vi "Error Create Queue.vi"(8 "error in (no error)":errorcluster) -> (0 "error out":errorcluster, 2 "Error Queue out":refnum<queue>, 3 "Error out":refnum<class "Error.lvclass">)   [LabVIEW 2019, in "TSC Error.lvlib"]
doc: "This VI will obtain a reference to the TSC Error Queue. If has not already been created, it will create the Queue.\n\nInputs:\n-error in\n\nOutputs:\n-Error out [obj] - the error class output\n-Error Queue out [Queue Ref] - a reference to the Error queue\n-error out\n________________________________________________________________________________\n<b>Code Developed By:</b>\nDaniel Coons\nTechnology Service Corporation\n1983 S Liberty Drive\nBloomington, IN 47403\nPhone: 812 558-7100\ndaniel.coons@tsc.com\nwww.tsc.com\n\n<b>Date Created:</b> 11 AUG 2014\n<b>Date Updated:</b>"
uses:
  TSC Error.lvlib
  _Messages/Error/Error.lvclass
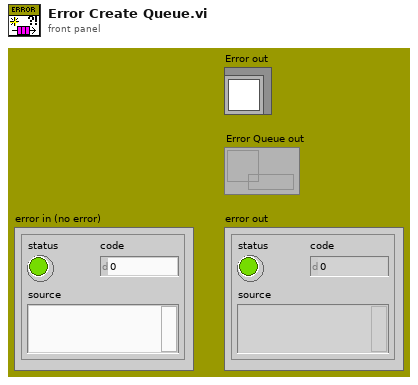
[diagram p1: front panel]
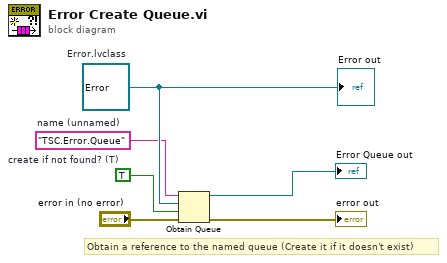
[diagram p0: block diagram]
diagram:
  w6 = refnum<class "Error.lvclass"> refnum  # Error.lvclass
  w5 = TRUE  # create if not found? (T)
  w3 = "TSC.Error.Queue"  # name (unnamed)
  # "Obtain a reference to the named queue (Create it if it doesn't exist)"
  n1 = Obtain Queue(name (unnamed)=w3, element data type=w6, create if not found? (T)=w5, error in (no error)="error in (no error)") -> (queue out=→"Error Queue out":refnum<queue>, error out=→"error out":errorcluster)  [unwired: 1 in, 1 out]
  "Error out" <- w6
